vi "runtime to editor crosslink test.vi"() -> (0 "error out":errorcluster, 2 "Pass":bool, 3 "Crosslinked?":bool)   [LabVIEW 2021, in "Multiplexer tests.lvlib"]
uses:
  Multiplexer tests.lvlib
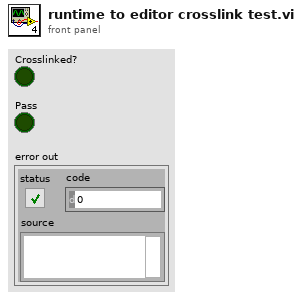
[diagram p1: front panel]
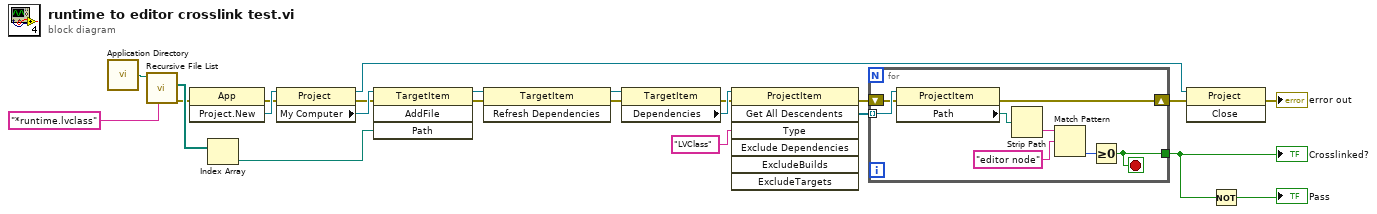
[diagram p0: block diagram]
diagram:
  n1 = call <vilib>:"Application Directory.vi"() -> ("Application Directory"=w7:path)
  n2 = call <vilib>:"Recursive File List.vi"("pattern"="*runtime.lvclass", "Folder Path"=w7) -> ("error out"=w3:errorcluster, "All Files in Dir"=w5:path[])  [unwired: 5 in, 3 out]
  n3 = invoke class="App" method="Project.New"(error in=w3) -> (error out=w17:errorcluster, "Project:New"=w20:refnum<vi>)  [unwired: 2 in, 1 out]
  n4 = Index Array(array=w5) -> (element=w4:path)  [unwired: 1 in]
  n5 = property class="Project"(reference=w20, error in=w17) -> (reference out=w11:refnum<vi>, error out=w18:errorcluster, "My Computer"=w19:refnum<vi>)
  n6 = invoke class="TargetItem" method="AddFile"(reference=w19, error in=w18, "Path"=w4) -> (reference out=w16:refnum<vi>, error out=w14:errorcluster)  [unwired: 1 in, 2 out]
  n7 = invoke class="TargetItem" method="Refresh Dependencies"(reference=w16, error in=w14) -> (reference out=w15:refnum<vi>, error out=w13:errorcluster)  [unwired: 1 in, 1 out]
  n8 = property class="TargetItem"(reference=w15, error in=w13) -> (error out=w9:errorcluster, "Dependencies"=w22:refnum<vi>)  [unwired: 1 out]
  n9 = invoke class="ProjectItem" method="Get All Descendents"(reference=w22, error in=w9, "Type"="LVClass") -> (error out=w10:errorcluster, "All Descendents"=w21:refnum<vi>[])  [unwired: 4 in, 5 out]
  n10 = for {
    tunnel: w21 -> [w31] mode=indexing
    shift-right: [w30] -> w12
    shift-left: w10 -> [w29]
    tunnel: [w24] -> w2
    stop <- w24 stop-if-true
    n11 = property class="ProjectItem"(reference=w31, error in=w29) -> (error out=w30:errorcluster, "Path"=w28:path)  [unwired: 1 out]
    n12 = Strip Path(path=w28) -> (name=w27:string)  [unwired: 1 out]
    n13 = Match Pattern(string=w27, regular expression="editor node") -> (offset past match=w25:i32)  [unwired: 1 in, 3 out]
    n14 = Greater Or Equal To 0?(x=w25) -> (x >= 0?=w24:bool)
  }
  "Crosslinked?" <- w2
  n15 = invoke class="Project" method="Close"(reference=w11, error in=w12) -> (error out=→"error out":errorcluster)  [unwired: 1 in, 2 out]
  n16 = Not(x=w2) -> (.not. x?=→"Pass":bool)
